vi "AH_SND.vi"(7 "Tries":i32=5, 8 "error in (no error)":errorcluster, 9 "CMD":string, 10 "Data Cluster In":T1 {"GUI Data Cluster"."SBR" format="%08b"}, 11 "Config Cluster In":T3={"General"={"Config.ini"=path "", "Default Logging Path"=path ""}, "Hardware"={"AHC VISA COM"="", "Measure Rate (1/s)"=0, "Global T VAR"="", "Global B VAR"="", "Average"=4, "Bias"=0, "Cable"={"Length"=0.0, "Resistance"=0.0, "Inductance"=0.0, "Capacitance"=0.0}, "Tracking"=0, "Voltage"=0.0}, "Operation"={"Operation Mode"=enum."Logging", "Status"="", "NewLog?"=FALSE}}) -> (0 "error IO":errorcluster, 2 "Data Cluster Out":T1 {"GUI Data Cluster"."SBR" format="%08b"}, 3 "Configuration Cluster Out":T3={"General"={"Config.ini"=path "", "Default Logging Path"=path ""}, "Hardware"={"AHC VISA COM"="", "Measure Rate (1/s)"=0, "Global T VAR"="", "Global B VAR"="", "Average"=4, "Bias"=0, "Cable"={"Length"=0.0, "Resistance"=0.0, "Inductance"=0.0, "Capacitance"=0.0}, "Tracking"=0, "Voltage"=0.0}, "Operation"={"Operation Mode"=enum."Idle-Off", "Status"="", "NewLog?"=FALSE}})   [LabVIEW 2021]
uses:
  Config_Cluster.ctl
  Mode_Enum.ctl
  Data_Cluster.ctl
  Measurement_Cluster.ctl
  Status_Byte.ctl
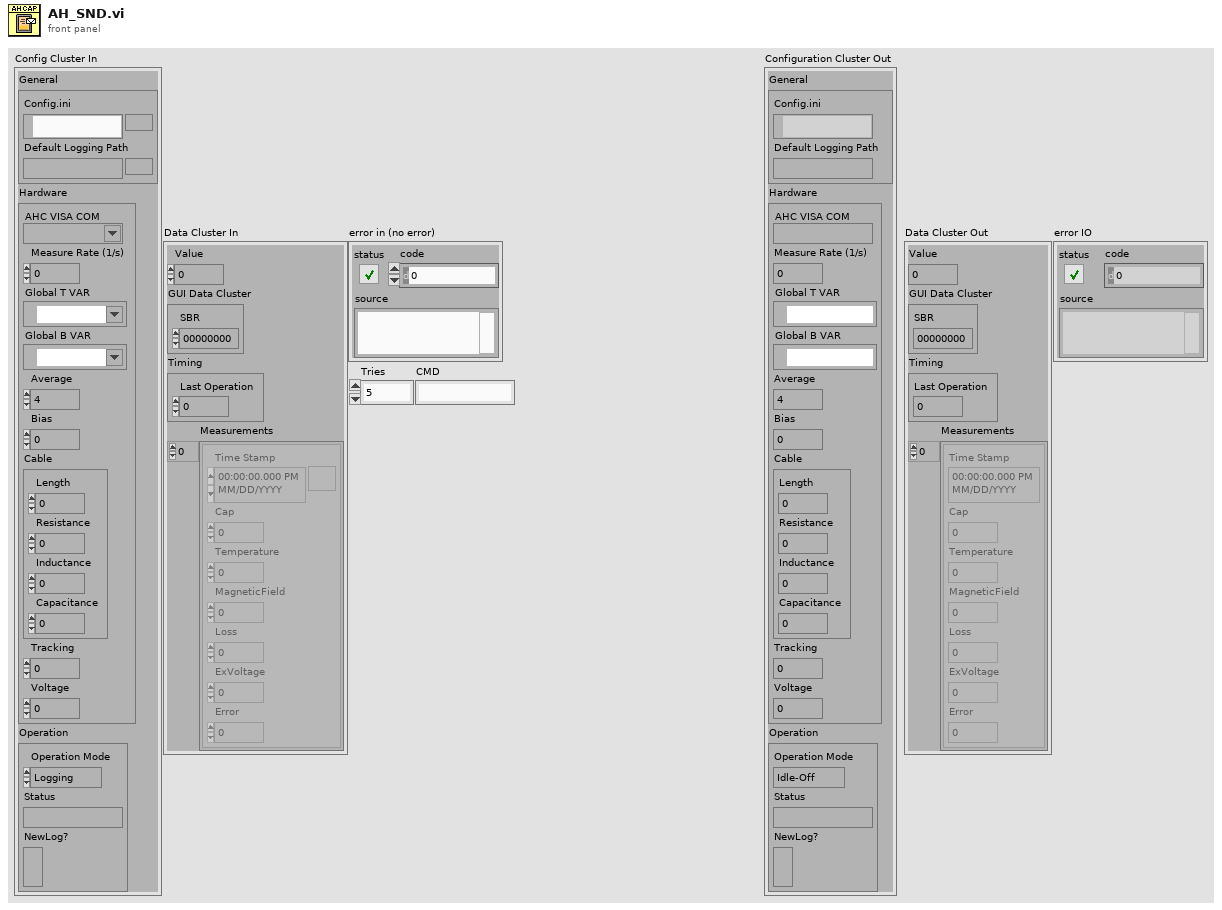
[diagram p1: front panel]
types:
  T1 = typedef "Data_Cluster.ctl" = cluster{"Value":dbl, "GUI Data Cluster":cluster{"SBR":u16}, "Timing":cluster{"Last Operation":dbl}, "Measurements":T2[]}
  T2 = typedef "Measurement_Cluster.ctl" = cluster{"Time Stamp":timestamp, "Cap":dbl, "Temperature":dbl, "MagneticField":dbl, "Loss":dbl, "ExVoltage":dbl, "Error":dbl}
  T3 = typedef "Config_Cluster.ctl" = cluster{"General":cluster{"Config.ini":path, "Default Logging Path":path}, "Hardware":cluster{"AHC VISA COM":refnum<visa-resource-name>, "Measure Rate (1/s)":i32, "Global T VAR":refnum<k21>, "Global B VAR":refnum<k21>, "Average":u8, "Bias":u8, "Cable":cluster{"Length":dbl, "Resistance":dbl, "Inductance":dbl, "Capacitance":dbl}, "Tracking":u8, "Voltage":dbl}, "Operation":cluster{"Operation Mode":T4, "Status":string, "NewLog?":bool}}
  T4 = typedef "Mode_Enum.ctl" = enum16{"Logging", "Idle-Off", "Idle"}
  T5 = typedef "Status_Byte.ctl" = u16
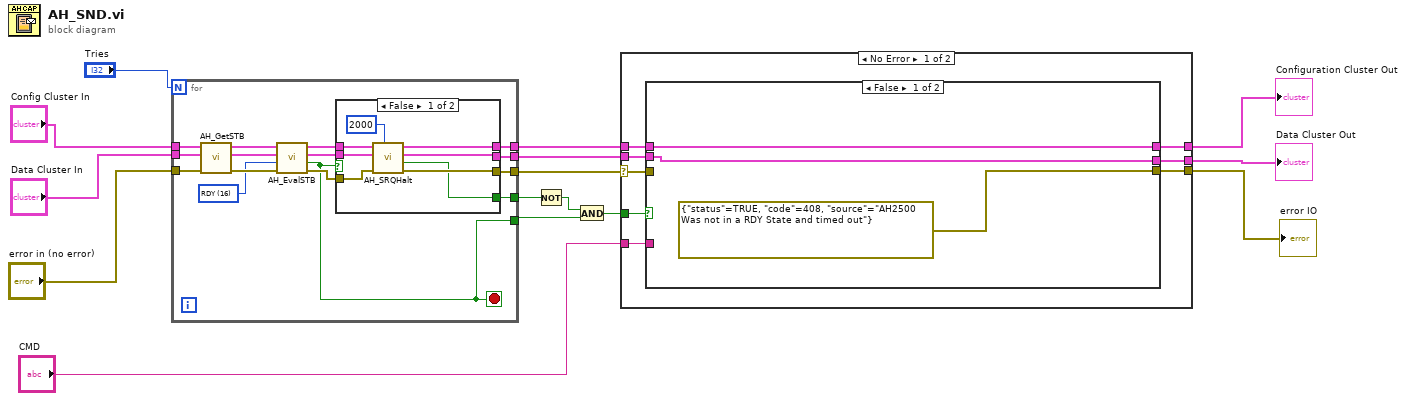
[diagram p0: block diagram]
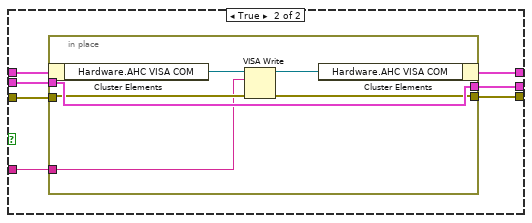
[diagram p2: hidden frame]
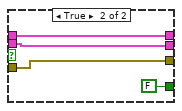
[diagram p4: hidden frame]
diagram:
  n1 = for {
    N: "Tries" -> [_]
    tunnel: "Config Cluster In" -> [w30]
    tunnel: "Data Cluster In" -> [w28]
    tunnel: "error in (no error)" -> [w27]
    tunnel: [w20] -> w7
    tunnel: [w19] -> w6
    tunnel: [w18] -> w8
    tunnel: [w17] -> w11
    tunnel: [w16] -> w9
    stop <- w16 stop-if-true
    w24 = T5 16 items=["ONR"=1, "CME"=2, "URQ"=4, "PON"=8, "RDY"=16, "EXE"=32, "RQS"=64, "MAV"=128] ("Status Byte")
    n2 = call "AH_GetSTB.vi"("error in (no error)"=w27, "Data Cluster In"=w28, "Config Cluster In"=w30) -> ("error out"=w25:errorcluster, "Data Cluster Out"=w26:T1, "Configuration Cluster Out"=w29:T3)  [unwired: 6 in]
    n3 = call "AH_EvalSTB.vi"("error in (no error)"=w25, "Status Byte"=w24, "Data Cluster In"=w26, "Config Cluster In"=w29) -> ("error out"=w21:errorcluster, "Result"=w16:bool, "Data Cluster Out"=w22:T1, "Configuration Cluster Out"=w23:T3)  [unwired: 3 in, 1 out]
    n4 = case shown="False" w16 {
      tunnel: w23 -> [w38 w42]
      tunnel: w22 -> [w36 w41]
      tunnel: w21 -> [w34 w40]
      tunnel: [w37 w42] -> w20
      tunnel: [w35 w41] -> w19
      tunnel: [w33 w40] -> w18
      tunnel: [w31 FALSE ("SRQ Timed Out")] -> w17
      frame False {
        n5 = call "AH_SRQHalt.vi"("timeout"=u32 2000, "error in (no error)"=w34, "Data Cluster In"=w36, "Config Cluster In"=w38) -> ("error out"=w33:errorcluster, "SRQ Timed Out"=w31:bool, "Data Cluster Out"=w35:T1, "Configuration Cluster Out"=w37:T3)  [unwired: 4 in]
      }
      frame True {
      }
    }
  }
  n6 = Not(x=w11) -> (.not. x?=w10:bool)
  n7 = And(x=w10, y=w9) -> (x .and. y?=w5:bool)
  n8 = case shown="No Error" w8 {
    selector: w8 -> [w47 w67]
    tunnel: w7 -> [w49 w69]
    tunnel: w6 -> [w48 w68]
    tunnel: w5 -> [w50 _]
    tunnel: [w46 w69] -> w3
    tunnel: [w45 w68] -> w2
    tunnel: [w44 w67] -> w1
    tunnel: "CMD" -> [w43 _]
    frame No Error {
      n9 = case shown="False" w50 {
        tunnel: w49 -> [w53 w60]
        tunnel: w48 -> [w52 w59]
        tunnel: w47 -> [_ w58]
        tunnel: [w53 w57] -> w46
        tunnel: [w52 w56] -> w45
        tunnel: [errorcluster {"status"=TRUE, "code"=408, "source"="AH2500 Was not in a RDY State and timed out"} ("error out") w55] -> w44
        tunnel: w43 -> [_ w54]
        frame False {
        }
        frame True {
          n10 = in-place {
            in-place-border: w59 -> [w64]
            in-place-border: w58 -> [w63]
            in-place-border: [w64] -> w56
            in-place-border: [w62] -> w55
            in-place-border: w54 -> [w61]
            n11 = in-place-cluster #1(w60) -> ("Hardware.AHC VISA COM"=w66:refnum<visa-resource-name>)
            n12 = VISA Write(VISA resource name=w66, write buffer=w61, error in (no error)=w63) -> (VISA resource name out=w65:refnum<visa-resource-name>, error out=w62:errorcluster)  [unwired: 1 out]
            n13 = in-place-cluster #1("Hardware.AHC VISA COM"=w65) -> (w57:T3)
          }
        }
      }
    }
    frame Error {
    }
  }
  "Configuration Cluster Out" <- w3
  "Data Cluster Out" <- w2
  "error IO" <- w1
